vi "Write Character.vi"(8 "error in (no error)":errorcluster, 10 "Character":u8 format="%.0x", 11 "Character in":refnum<class "Character.lvclass">) -> (0 "error out":errorcluster, 3 "Character out":refnum<class "Character.lvclass">)   [LabVIEW 2016, in "Character.lvclass"]
uses:
  Character.lvclass
  Character.lvclass/Character.ctl
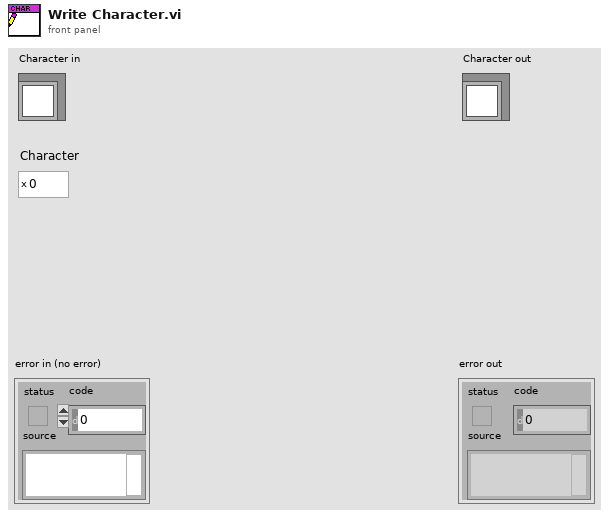
[diagram p1: front panel]
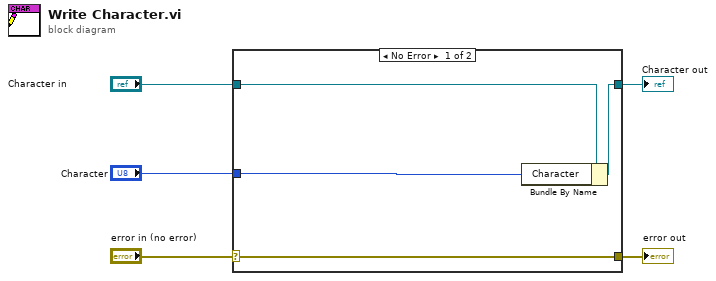
[diagram p0: block diagram]
diagram:
  n1 = case shown="No Error" "error in (no error)" {
    selector: "error in (no error)" -> [w9 w10]
    tunnel: [w9 w10] -> w4
    tunnel: [w7 w11] -> w2
    tunnel: "Character in" -> [w8 w11]
    tunnel: "Character" -> [w6 _]
    frame No Error {
      n2 = Bundle By Name(cluster=w8, "Character"=w6) -> (w7:refnum<class "Character.lvclass">)
    }
    frame Error {
    }
  }
  "error out" <- w4
  "Character out" <- w2
